vi "Configure Limit Testing.vi"(0 "VISA resource name":refnum<visa-resource-name>, 1 "Limit (1: Limit 1)":i32(ring)=1 items=["Limit 1"=1, "Limit 2"=2], 5 "Enable Limit Test (F: Disable)":bool, 7 "Autoclear Limit (T: Enable)":bool=TRUE, 9 "Upper Limit (1)":dbl=1.0, 11 "error in (no error)":errorcluster, 12 "Lower Limit (-1)":dbl=-1.0) -> (4 "VISA resource name out":refnum<visa-resource-name>, 15 "error out":errorcluster)   [LabVIEW 2020, in "Keithley 2182.lvlib"]
doc: "Configures limit testing.\n\nLimit operations set and control the values that determine the HI/IN/LO status of subsequent\nmeasurements. The limit test is performed on the result of an enabled Rel, mX+b, or Percent\noperation.\n\nThere are two sets of limits. Limit 1 uses high and low limits (HI1 and LO1) as does Limit 2\n(HI2 and LO2). However, the HI/IN/LO status message only applies to Limit 1. The figure below illustrates the following limits, which are factory defaults:\n<B>Limit 1: HI1 = +1V and LO1 = -1V\nLimit 2: HI2 = +2V and LO2 = -2V</B>\n\n<--------LO--------X--------IN--------X--------HI-------->\n<----------------------------------------------------------->\n | | | | |\n -2V -1V 0 1V 2V\n LO2 LO1 HI1 HI2 \n | | | |\n | -----Limit 1------- |\n ----------------Limit 2----------------"
uses:
  Keithley 2182.lvlib
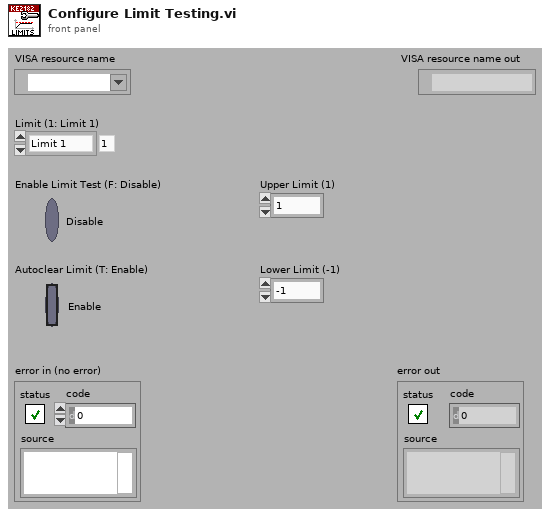
[diagram p1: front panel]
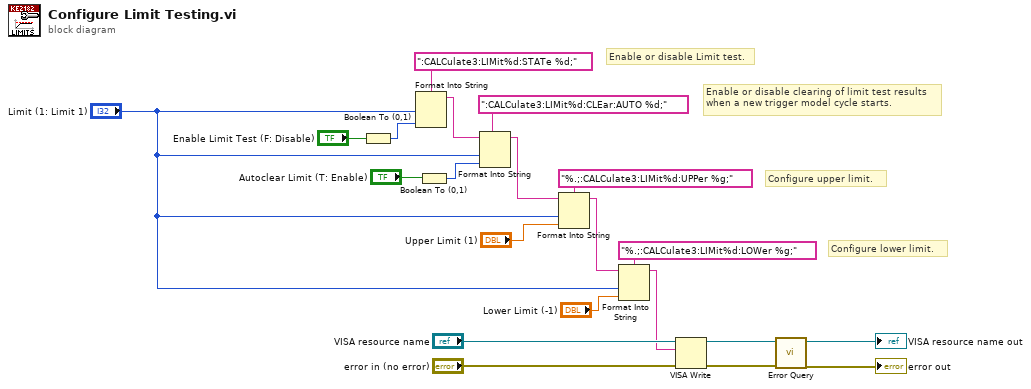
[diagram p0: block diagram]
diagram:
  # "Configure lower limit."
  # "Configure upper limit."
  # "Enable or disable clearing of limit test results\nwhen a new trigger model cycle starts."
  # "Enable or disable Limit test."
  n1 = Boolean To (0,1)(Boolean="Enable Limit Test (F: Disable)") -> (0, 1=w11:i16)
  n2 = Format Into String(format string=":CALCulate3:LIMit%d:STATe %d;", "Limit (1: Limit 1)", w11) -> (resulting string=w1:string)  [unwired: 2 in, 1 out]
  n3 = Boolean To (0,1)(Boolean="Autoclear Limit (T: Enable)") -> (0, 1=w8:i16)
  n4 = Format Into String(format string=":CALCulate3:LIMit%d:CLEar:AUTO %d;", initial string=w1, "Limit (1: Limit 1)", w8) -> (resulting string=w2:string)  [unwired: 1 in, 1 out]
  n5 = Format Into String(format string="%.;:CALCulate3:LIMit%d:UPPer %g;", initial string=w2, "Limit (1: Limit 1)", "Upper Limit (1)") -> (resulting string=w3:string)  [unwired: 1 in, 1 out]
  n6 = Format Into String(format string="%.;:CALCulate3:LIMit%d:LOWer %g;", initial string=w3, "Limit (1: Limit 1)", "Lower Limit (-1)") -> (resulting string=w4:string)  [unwired: 1 in, 1 out]
  n7 = VISA Write(VISA resource name="VISA resource name", write buffer=w4, error in (no error)="error in (no error)") -> (VISA resource name out=w17:refnum<visa-resource-name>, error out=w16:errorcluster)  [unwired: 1 out]
  n8 = call "Error Query.vi"("error in (no error)"=w16, "VISA resource name"=w17) -> ("error out"=→"error out":errorcluster, "VISA resource name out"=→"VISA resource name out":refnum<visa-resource-name>)  [unwired: 6 in, 2 out]
